vi "5.2.2.-Detección de Bordes y Suavizado Gaussiano.vi"(10 "CAPA DE COLOR":T1) -> ()   [LabVIEW 2020]
uses:
  5.2.0.-ENUM Capas RGB y HSV de Imagen.ctl
  <vilib>/Math Plots/3D Math Plots/3D Mesh/3D Mesh XCtrl/3D Mesh.xctl
  <vilib>/Math Plots/3D Math Plots/3D Mesh/3D Mesh Datatype/Public/Plot Helper (Matrix).vi
  <vilib>/Math Plots/3D Math Plots/3D Mesh/3D Mesh Datatype/3D Mesh Datatype.lvclass
  <vilib>/vision/NI_Vision_Development_Module.lvlib
panel:
  out "Capa de color de imagen original":picture
  out "J":i32[][](array[numeric])
  out "Mesh":refnum<class "3D Plot Datatype.lvclass">[](xcontrol)
  out "Phi":dbl[][](array[numeric])
  out "G":dbl[][](array[numeric])
  out "Bordes de imagen después de suavizado":picture
  out "h":dbl[][](array[numeric])
  in  "sigma":dbl
  in  "T":dbl
  in  "Seleccionar Imagen":path
  # "Visión Artificial - Suavizado de Imagen - Filtro Gaussiano\nDiego Cervantes Rodríguez\ndicer0.com"
  # "Suavizado con Filtro Gaussiano"
  # "Gradiente de Filtro Gaussiano"
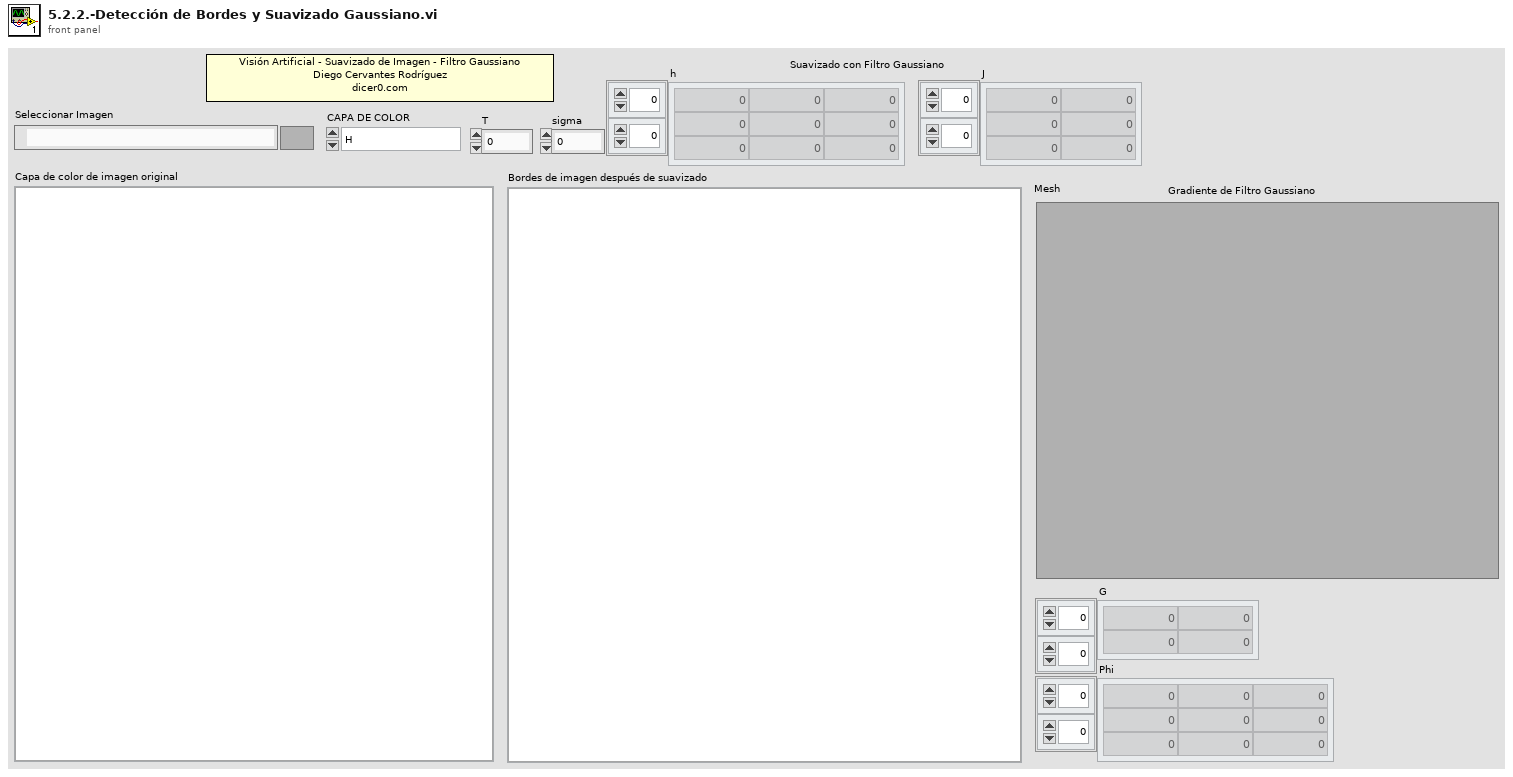
[diagram p1: front panel]
types:
  T1 = typedef "5.2.0.-ENUM Capas RGB y HSV de Imagen.ctl" = enum16{"H", "S", "V", "R", "G", "B", "RGB2GRAY MATLAB"}
  T2 = typedef "imagedata.ctl" = cluster{"image type":i32, "image depth":i32, "image":u8[], "mask":u8[], "colors":u32[], "Rectangle":cluster{"left":i16, "top":i16, "right":i16, "bottom":i16}}
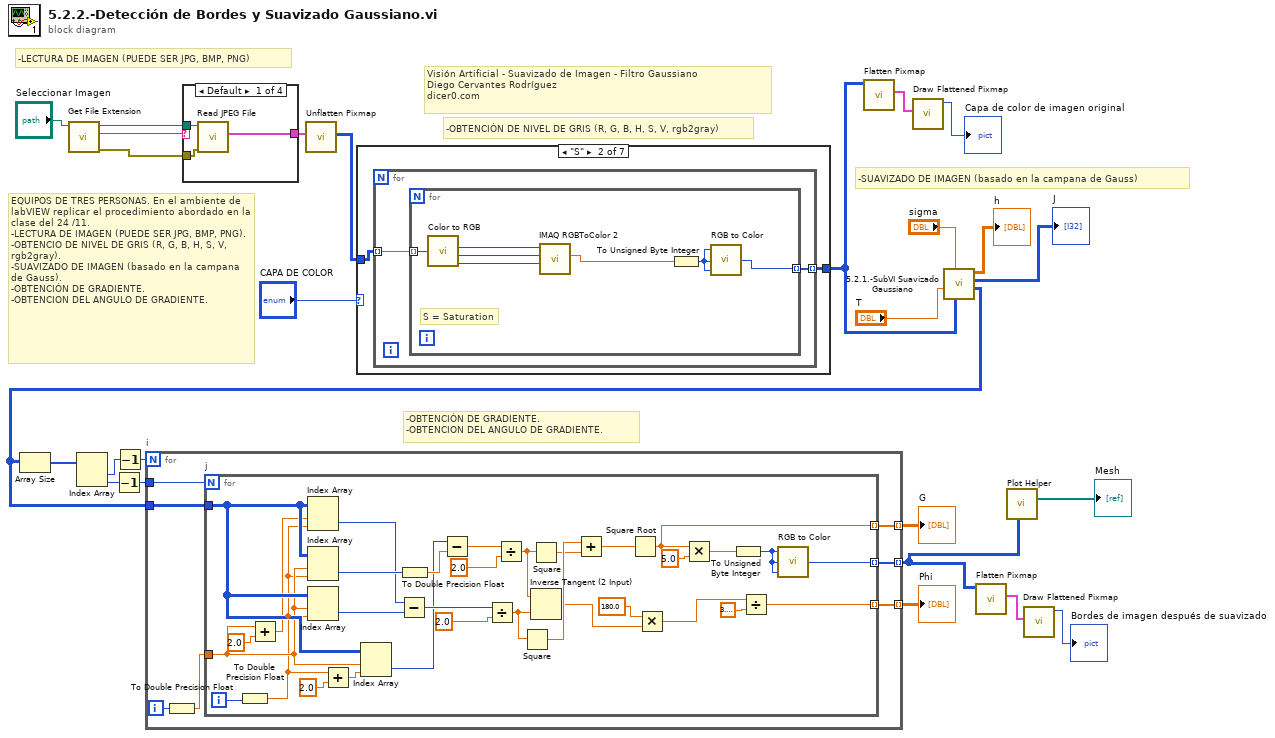
[diagram p0: block diagram]
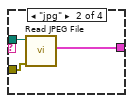
[diagram p2: hidden frame]
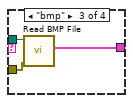
[diagram p3: hidden frame]
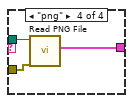
[diagram p4: hidden frame]
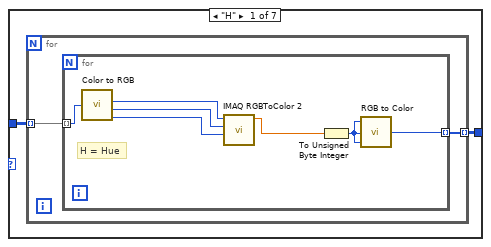
[diagram p5: hidden frame]
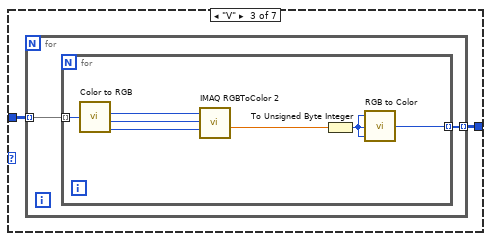
[diagram p6: hidden frame]
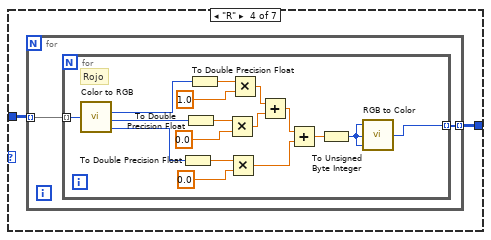
[diagram p7: hidden frame]
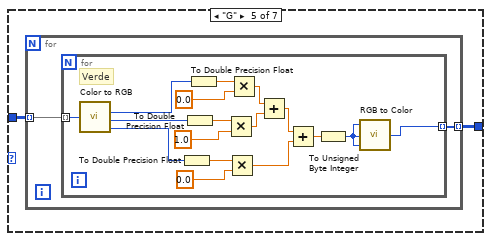
[diagram p8: hidden frame]
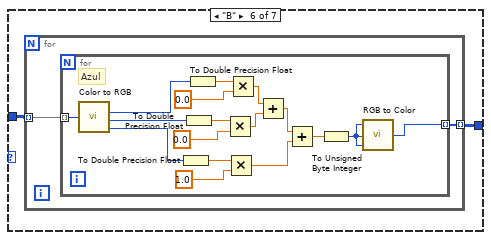
[diagram p9: hidden frame]
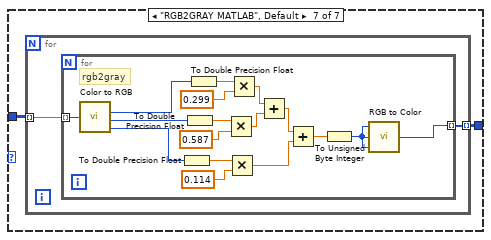
[diagram p10: hidden frame]
diagram:
  # "Visión Artificial - Suavizado de Imagen - Filtro Gaussiano\nDiego Cervantes Rodríguez\ndicer0.com"
  # "-SUAVIZADO DE IMAGEN (basado en la campana de Gauss)"
  # "-OBTENCIÓN DE GRADIENTE.\n-OBTENCION DEL ANGULO DE GRADIENTE."
  # "-OBTENCIÓN DE NIVEL DE GRIS (R, G, B, H, S, V, rgb2gray)"
  # "-LECTURA DE IMAGEN (PUEDE SER JPG, BMP, PNG)"
  # "EQUIPOS DE TRES PERSONAS. En el ambiente de labVIEW replicar el procedimiento abordado en la clase del 24 /11.\n-LECTURA DE IMAGEN (PUEDE SER JPG, BMP, PNG).\n-OBTENCIO DE NIVEL DE GRIS (R, G, B, H, S, V, rgb2gray).\n-SUAVIZADO DE IMAGEN (basado en la campana de Gauss).\n-OBTENCIÓN DE GRADIENTE.\n-OBTENCION DEL ANGULO DE GRADIENTE."
  n1 = call <vilib>:"Get File Extension.vi"("file"="Seleccionar Imagen") -> ("error out"=w24:errorcluster, "lowercase file extension"=w22:string, "dup file"=w23:path)  [unwired: 6 in, 2 out]
  n2 = case shown="Default" w22 {
    tunnel: w23 -> [w29 w32 w35 w38]
    tunnel: w24 -> [w28 w31 w34 w37]
    tunnel: [w27 w30 w33 w36] -> w20
    frame Default {
      n3 = call <vilib>:"Read JPEG File.vi"("error in (no error)"=w28, "path to JPEG file"=w29) -> ("image data"=w27:T2)  [unwired: 7 in, 2 out]
    }
    frame "jpg" {
      n4 = call <vilib>:"Read JPEG File.vi"("error in (no error)"=w31, "path to JPEG file"=w32) -> ("image data"=w30:T2)  [unwired: 7 in, 2 out]
    }
    frame "bmp" {
      n5 = call <vilib>:"Read BMP File.vi"("error in (no error)"=w34, "path to BMP file"=w35) -> ("image data"=w33:T2)  [unwired: 7 in, 2 out]
    }
    frame "png" {
      n6 = call <vilib>:"Read PNG File.vi"("error in (no error)"=w37, "path to PNG file"=w38) -> ("image data"=w36:T2)  [unwired: 7 in, 2 out]
    }
  }
  n7 = call <vilib>:"Unflatten Pixmap.vi"("image data"=w20) -> ("24-bit pixmap"=w26:u32[][])  [unwired: 4 in, 6 out]
  n8 = case shown="\"S\"" "CAPA DE COLOR" {
    tunnel: [w40 w50 w62 w72 w93 w114 w135] -> w4
    tunnel: w26 -> [w39 w51 w61 w73 w94 w115 w136]
    frame "H" {
      n9 = for {
        tunnel: w39 -> [w42] mode=indexing
        tunnel: [w41] -> w40 mode=indexing
        n10 = for {
          tunnel: w42 -> [w49] mode=indexing
          tunnel: [w47] -> w41 mode=indexing
          # "H = Hue"
          n11 = call <vilib>:"Color to RGB.vi"("Color"=w49) -> ("R"=w45:u8, "G"=w44:u8, "B"=w43:u8)  [unwired: 1 out]
          n12 = call "IMAQ RGBToColor 2"("Blue value"=w43, "Green value"=w44, "Red value"=w45) -> ("Red or Hue or X or L* value"=w46:dbl)  [unwired: 5 in, 3 out]
          n13 = To Unsigned Byte Integer(number=w46) -> (unsigned 8bit integer=w48:u8)
          n14 = call <vilib>:"RGB to Color.vi"("B"=w48, "G"=w48, "R"=w48) -> ("Color"=w47:u32)
        }
      }
    }
    frame "S" {
      n15 = for {
        tunnel: w51 -> [w53] mode=indexing
        tunnel: [w52] -> w50 mode=indexing
        n16 = for {
          tunnel: w53 -> [w60] mode=indexing
          tunnel: [w58] -> w52 mode=indexing
          # "S = Saturation"
          n17 = call <vilib>:"Color to RGB.vi"("Color"=w60) -> ("R"=w56:u8, "G"=w55:u8, "B"=w54:u8)  [unwired: 1 out]
          n18 = call "IMAQ RGBToColor 2"("Blue value"=w54, "Green value"=w55, "Red value"=w56) -> ("Green or Sat or Y or a* value"=w57:dbl)  [unwired: 5 in, 3 out]
          n19 = To Unsigned Byte Integer(number=w57) -> (unsigned 8bit integer=w59:u8)
          n20 = call <vilib>:"RGB to Color.vi"("B"=w59, "G"=w59, "R"=w59) -> ("Color"=w58:u32)
        }
      }
    }
    frame "V" {
      n21 = for {
        tunnel: w61 -> [w64] mode=indexing
        tunnel: [w63] -> w62 mode=indexing
        n22 = for {
          tunnel: w64 -> [w71] mode=indexing
          tunnel: [w69] -> w63 mode=indexing
          n23 = call <vilib>:"Color to RGB.vi"("Color"=w71) -> ("R"=w68:u8, "G"=w67:u8, "B"=w66:u8)  [unwired: 1 out]
          n24 = call "IMAQ RGBToColor 2"("Blue value"=w66, "Green value"=w67, "Red value"=w68) -> ("Blue or Luma or Val or Inten or Z or b*value"=w65:dbl)  [unwired: 5 in, 3 out]
          n25 = To Unsigned Byte Integer(number=w65) -> (unsigned 8bit integer=w70:u8)
          n26 = call <vilib>:"RGB to Color.vi"("B"=w70, "G"=w70, "R"=w70) -> ("Color"=w69:u32)
        }
      }
    }
    frame "R" {
      n27 = for {
        tunnel: w73 -> [w75] mode=indexing
        tunnel: [w74] -> w72 mode=indexing
        n28 = for {
          tunnel: w75 -> [w92] mode=indexing
          tunnel: [w87] -> w74 mode=indexing
          # "Rojo"
          n29 = call <vilib>:"Color to RGB.vi"("Color"=w92) -> ("R"=w86:u8, "G"=w84:u8, "B"=w82:u8)  [unwired: 1 out]
          n30 = To Double Precision Float(number=w82) -> (double precision float=w81:dbl)
          n31 = To Double Precision Float(number=w84) -> (double precision float=w83:dbl)
          n32 = To Double Precision Float(number=w86) -> (double precision float=w85:dbl)
          n33 = Multiply(x=w83, y=0.0) -> (x*y=w78:dbl)
          n34 = Multiply(x=w81, y=0.0) -> (x*y=w79:dbl)
          n35 = Multiply(x=w85, y=1.0) -> (x*y=w77:dbl)
          n36 = Add(x=w77, y=w78) -> (x+y=w80:dbl)
          n37 = Add(x=w80, y=w79) -> (x+y=w76:dbl)
          n38 = To Unsigned Byte Integer(number=w76) -> (unsigned 8bit integer=w88:u8)
          n39 = call <vilib>:"RGB to Color.vi"("B"=w88, "G"=w88, "R"=w88) -> ("Color"=w87:u32)
        }
      }
    }
    frame "G" {
      n40 = for {
        tunnel: w94 -> [w96] mode=indexing
        tunnel: [w95] -> w93 mode=indexing
        n41 = for {
          tunnel: w96 -> [w113] mode=indexing
          tunnel: [w108] -> w95 mode=indexing
          # "Verde"
          n42 = call <vilib>:"Color to RGB.vi"("Color"=w113) -> ("R"=w107:u8, "G"=w105:u8, "B"=w103:u8)  [unwired: 1 out]
          n43 = To Double Precision Float(number=w103) -> (double precision float=w102:dbl)
          n44 = To Double Precision Float(number=w105) -> (double precision float=w104:dbl)
          n45 = To Double Precision Float(number=w107) -> (double precision float=w106:dbl)
          n46 = Multiply(x=w104, y=1.0) -> (x*y=w99:dbl)
          n47 = Multiply(x=w102, y=0.0) -> (x*y=w100:dbl)
          n48 = Multiply(x=w106, y=0.0) -> (x*y=w98:dbl)
          n49 = Add(x=w98, y=w99) -> (x+y=w101:dbl)
          n50 = Add(x=w101, y=w100) -> (x+y=w97:dbl)
          n51 = To Unsigned Byte Integer(number=w97) -> (unsigned 8bit integer=w109:u8)
          n52 = call <vilib>:"RGB to Color.vi"("B"=w109, "G"=w109, "R"=w109) -> ("Color"=w108:u32)
        }
      }
    }
    frame "B" {
      n53 = for {
        tunnel: w115 -> [w117] mode=indexing
        tunnel: [w116] -> w114 mode=indexing
        n54 = for {
          tunnel: w117 -> [w134] mode=indexing
          tunnel: [w129] -> w116 mode=indexing
          # "Azul"
          n55 = call <vilib>:"Color to RGB.vi"("Color"=w134) -> ("R"=w128:u8, "G"=w126:u8, "B"=w124:u8)  [unwired: 1 out]
          n56 = To Double Precision Float(number=w124) -> (double precision float=w123:dbl)
          n57 = To Double Precision Float(number=w126) -> (double precision float=w125:dbl)
          n58 = To Double Precision Float(number=w128) -> (double precision float=w127:dbl)
          n59 = Multiply(x=w125, y=0.0) -> (x*y=w120:dbl)
          n60 = Multiply(x=w123, y=1.0) -> (x*y=w121:dbl)
          n61 = Multiply(x=w127, y=0.0) -> (x*y=w119:dbl)
          n62 = Add(x=w119, y=w120) -> (x+y=w122:dbl)
          n63 = Add(x=w122, y=w121) -> (x+y=w118:dbl)
          n64 = To Unsigned Byte Integer(number=w118) -> (unsigned 8bit integer=w130:u8)
          n65 = call <vilib>:"RGB to Color.vi"("B"=w130, "G"=w130, "R"=w130) -> ("Color"=w129:u32)
        }
      }
    }
    frame "RGB2GRAY MATLAB", Default {
      n66 = for {
        tunnel: w136 -> [w138] mode=indexing
        tunnel: [w137] -> w135 mode=indexing
        n67 = for {
          tunnel: w138 -> [w155] mode=indexing
          tunnel: [w150] -> w137 mode=indexing
          # "rgb2gray"
          n68 = call <vilib>:"Color to RGB.vi"("Color"=w155) -> ("R"=w149:u8, "G"=w147:u8, "B"=w145:u8)  [unwired: 1 out]
          n69 = To Double Precision Float(number=w145) -> (double precision float=w144:dbl)
          n70 = To Double Precision Float(number=w147) -> (double precision float=w146:dbl)
          n71 = To Double Precision Float(number=w149) -> (double precision float=w148:dbl)
          n72 = Multiply(x=w146, y=0.587) -> (x*y=w141:dbl)
          n73 = Multiply(x=w144, y=0.114) -> (x*y=w142:dbl)
          n74 = Multiply(x=w148, y=0.299) -> (x*y=w140:dbl)
          n75 = Add(x=w140, y=w141) -> (x+y=w143:dbl)
          n76 = Add(x=w143, y=w142) -> (x+y=w139:dbl)
          n77 = To Unsigned Byte Integer(number=w139) -> (unsigned 8bit integer=w151:u8)
          n78 = call <vilib>:"RGB to Color.vi"("B"=w151, "G"=w151, "R"=w151) -> ("Color"=w150:u32)
        }
      }
    }
  }
  n79 = call <vilib>:"Flatten Pixmap.vi"("24-bit pixmap"=w4) -> ("image data"=w6:T2)  [unwired: 10 in]
  n80 = call <vilib>:"Draw Flattened Pixmap.vi"("image data"=w6) -> ("new picture"=→"Capa de color de imagen original":picture)  [unwired: 8 in]
  n81 = call "5.2.1.-SubVI Suavizado Gaussiano.vi"("Capa de color"=w4, "Sigma"="sigma", "T"="T") -> ("Array out"=w1:i32[][], "J"=→"J":i32[][], "h"=→"h":dbl[][])  [unwired: 6 in]
  n82 = Array Size(array=w1) -> (size(s)=w17:i32[])
  n83 = Index Array "Index Array"(array=w17) -> (element #1=w16:i32, element #2=w14:i32)  [unwired: 2 in]
  n84 = Decrement(x=w14) -> (x-1=w13:i32)
  n85 = Decrement(x=w16) -> (x-1=w15:i32)
  n86 = for "i" {
    N: w15 -> [_]
    tunnel: w13 -> [w162]
    tunnel: w1 -> [w161]
    tunnel: [w160] -> w8 mode=indexing
    tunnel: [w159] -> w7 mode=indexing
    tunnel: [w158] -> w10 mode=indexing
    i -> [w157]
    n87 = To Double Precision Float(number=w157) -> (double precision float=w156:dbl)
    n88 = for "j" {
      N: w162 -> [_]
      tunnel: w156 -> [w191]
      tunnel: w161 -> [w193]
      tunnel: [w177] -> w160 mode=indexing
      tunnel: [w178] -> w159 mode=indexing
      tunnel: [w168] -> w158 mode=indexing
      i -> [w167]
      n89 = To Double Precision Float(number=w167) -> (double precision float=w166:dbl)
      n90 = Add(x=w191, y=2.0) -> (x+y=w192:dbl)
      n91 = Index Array "Index Array"(array=w193, index (row)=w192, index (col)=w166) -> (element=w163:i32)
      n92 = Index Array(array=w193, index (row)=w191, index (col)=w166) -> (element=w188:i32)
      n93 = Index Array(array=w193, index (row)=w191, index (col)=w166) -> (element=w164:i32)
      n94 = Add(x=w166, y=2.0) -> (x+y=w189:dbl)
      n95 = Index Array(array=w193, index (row)=w191, index (col)=w189) -> (element=w165:i32)
      n96 = Subtract(x=w163, y=w164) -> (x-y=w186:i32)
      n97 = To Double Precision Float(number=w188) -> (double precision float=w187:dbl)
      n98 = Subtract(x=w165, y=w187) -> (x-y=w183:dbl)
      n99 = Divide(x=w186, y=2.0) -> (x/y=w174:dbl)
      n100 = Divide(x=w183, y=2.0) -> (x/y=w173:dbl)
      n101 = Square(x=w174) -> (x^2=w182:dbl)
      n102 = Square(x=w173) -> (x^2=w181:dbl)
      n103 = Inverse Tangent (2 Input)(1:w174, 2:w173) -> (0:w172:dbl)
      n104 = Add(x=w182, y=w181) -> (x+y=w180:dbl)
      n105 = Square Root(x=w180) -> (sqrt(x)=w177:dbl)
      n106 = Multiply(x=180.0, y=w172) -> (x*y=w170:dbl)
      n107 = Multiply(x=w177, y=5.0) -> (x*y=w175:dbl)
      n108 = To Unsigned Byte Integer(number=w175) -> (unsigned 8bit integer=w179:u8)
      n109 = Divide(x=w170, y=3.141592653589793) -> (x/y=w168:dbl)
      n110 = call <vilib>:"RGB to Color.vi"("B"=w179, "G"=w179, "R"=w179) -> ("Color"=w178:u32)
    }
  }
  "G" <- w8
  "Phi" <- w10
  n111 = call <vilib>:"Flatten Pixmap.vi"("24-bit pixmap"=w7) -> ("image data"=w12:T2)  [unwired: 10 in]
  n112 = call-poly <vilib>:"Plot Helper.vi"("z matrix"=w7) -> ("3D Plot lvclass Array out"=→"Mesh":refnum<class "3D Plot Datatype.lvclass">[])  [unwired: 5 in, 5 out]
  n113 = call <vilib>:"Draw Flattened Pixmap.vi"("image data"=w12) -> ("new picture"=→"Bordes de imagen después de suavizado":picture)  [unwired: 8 in]
